vi "uTransport_Destroy.vi"(8 "error in (no error)":errorcluster, 11 "uActor in":refnum<class "uActor.lvclass">) -> (0 "error out":errorcluster)   [LabVIEW 2023, in "uLib.lvlib" / "uActor.lvclass"]
doc: "Invoking this method on an actor does not immediately destroy it, instead it enqueues a self-stop message that takes its turn in the actor's internal FIFO queue.\n\nThis method executes regardless of the error-in state."
uses:
  uActor.lvclass
  uActor.lvclass/uActor.ctl
  uMsg/uMsg/uMsg.lvclass/uMsg.ctl
  uTransport/uTransport_uActor/uTransport_uActor.lvclass/uTransport_uActor.ctl
  uActor_CMDs_Prefix.vi
  uActor_SimpleSend.vi
  uActor_SendMsg.vi
  uMsg/uMsg/uMsg Create.vi
  uTransport/uTransport_uActor/uTransport_uActor_SendMsg.vi
  uMsg/uMsg/uMsg Update Timestamp.vi
  uData/uData/uData.lvclass
  uTransport/uTransport/uTransport.lvclass
  uMsg/uMsg/uMsg.lvclass
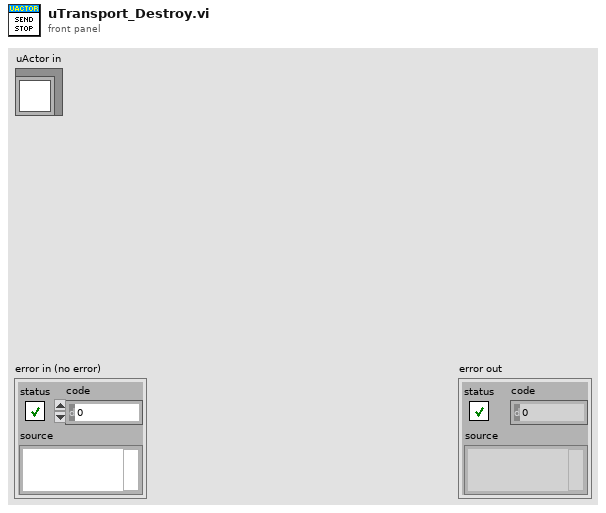
[diagram p1: front panel]
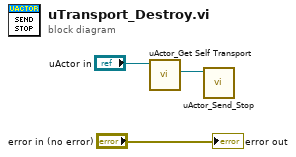
[diagram p0: block diagram]
diagram:
  n1 = call "uActor_Get Self Transport.vi"("uActor in"="uActor in") -> ("Actor Transport"=w1:refnum<class "uTransport_uActor.lvclass">)  [unwired: 9 in, 1 out]
  n2 = call "uActor_Send_Stop.vi"("uActor Transport"=w1) -> ()  [unwired: 10 in, 1 out]
  "error out" <- "error in (no error)"
